vi "Set Enabled State.vi"(8 "error in (no error)":errorcluster, 10 "Enabled?":bool, 11 "Log Sink":refnum<data-value>) -> (0 "error out":errorcluster)   [LabVIEW 2018, in "MVA Framework.lvlib" / "Composed Log.lvlib" / "Log Sink.lvclass"]
uses:
  Log Sink.lvclass
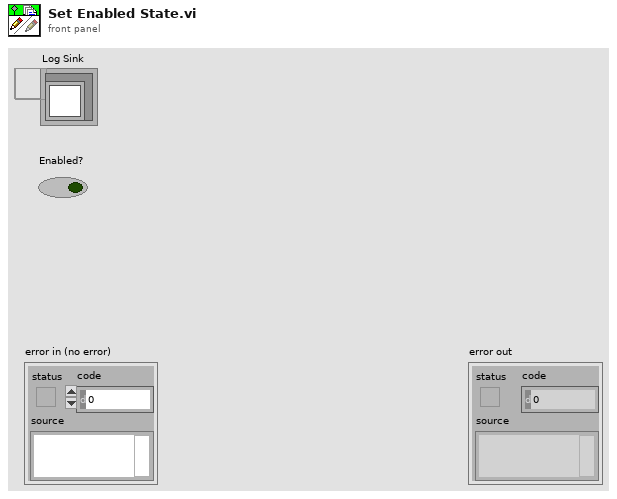
[diagram p1: front panel]
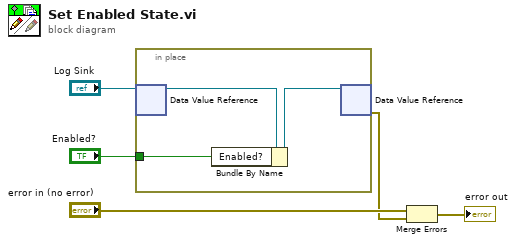
[diagram p0: block diagram]
diagram:
  n1 = in-place {
    in-place-border: "Enabled?" -> [w6]
    n2 = in-place-dvr #1("Log Sink") -> (w8:refnum<class "Log Sink.lvclass">)  [unwired: 1 out]
    n3 = Bundle By Name(cluster=w8, "Enabled?"=w6) -> (w7:refnum<class "Log Sink.lvclass">)
    n4 = in-place-dvr #1(w7) -> (w2:errorcluster)  [unwired: 1 out]
  }
  n5 = Merge Errors("error in (no error)", w2) -> (→"error out":errorcluster)
